vi "VLC-IP_FGV_param.vi"(9 "SamplingTime_in":i32, 10 "Mode":enum16{"Read", "Write"}(ring), 11 "TemporaryFilePath_in":path) -> (2 "SamplingTime_out":i32, 3 "TemporaryFilePath_out":path)   [LabVIEW 2016]
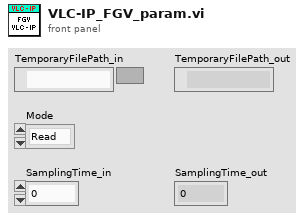
[diagram p1: front panel]
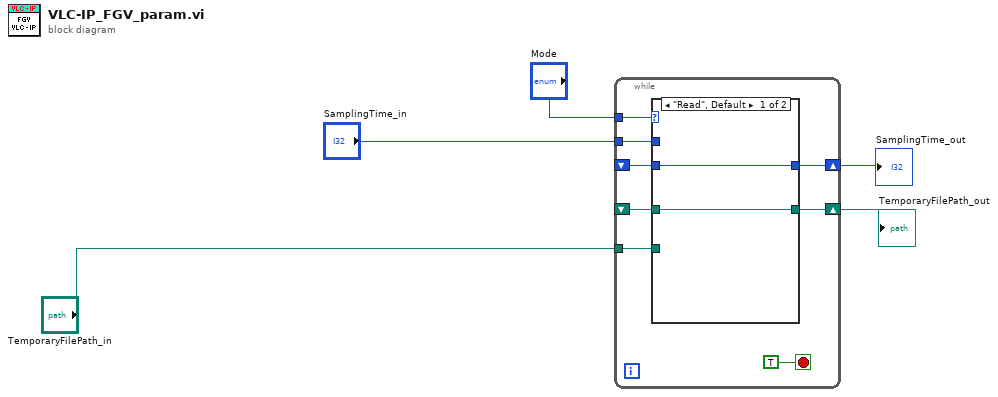
[diagram p0: block diagram]
diagram:
  n1 = while {
    tunnel: "Mode" -> [w12]
    tunnel: "SamplingTime_in" -> [w10]
    shift-right: [w11] -> w3
    shift-left: _ -> [w9]
    tunnel: "TemporaryFilePath_in" -> [w7]
    shift-right: [w8] -> w5
    shift-left: _ -> [w6]
    stop <- TRUE stop-if-true
    n2 = case shown="\"Read\", Default" w12 {
      tunnel: [w15 w17] -> w11
      tunnel: w10 -> [_ w17]
      tunnel: w9 -> [w15 _]
      tunnel: [w14 w16] -> w8
      tunnel: w7 -> [_ w16]
      tunnel: w6 -> [w14 _]
      frame "Read", Default {
      }
      frame "Write" {
      }
    }
  }
  "TemporaryFilePath_out" <- w5
  "SamplingTime_out" <- w3
